vi "TDC_getCoincCounters.vi"(8 "Error In":errorcluster) -> (0 "Error Out":errorcluster, 1 "Update Count":i32, 2 "Penta Coincidences":i32, 3 "Quad Coincidences":i32[](array[numeric]), 5 "Triple Coincidences":i32[](array[numeric]), 7 "Pair Coincidences":i32[](array[numeric]), 11 "Single Counts":i32[](array[numeric]))   [LabVIEW 2011]
uses:
  tdcbase.dll
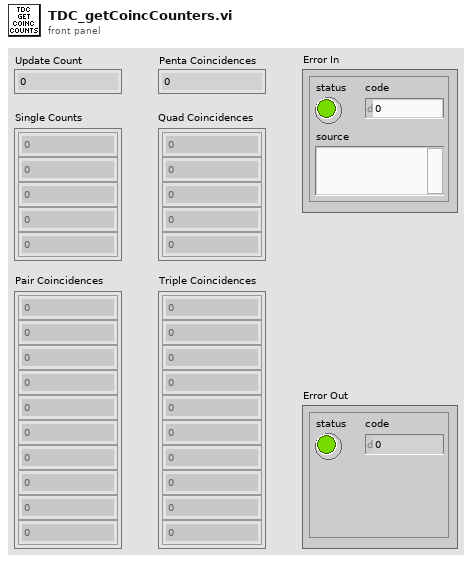
[diagram p1: front panel]
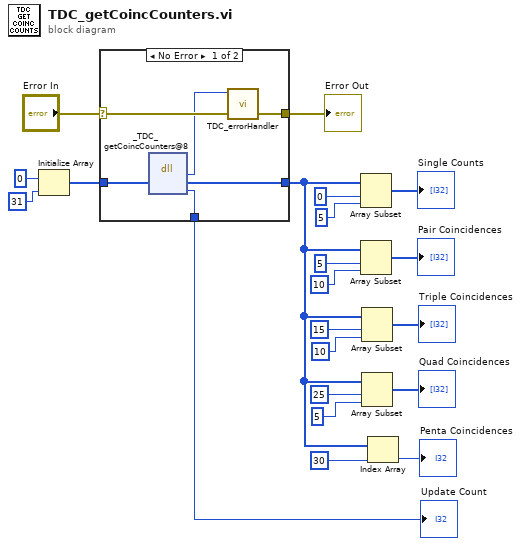
[diagram p0: block diagram]
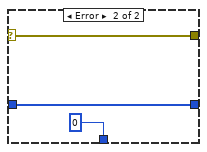
[diagram p2: hidden frame]
diagram:
  n1 = Initialize Array(0, 31) -> (w1:i32[])
  n2 = case shown="No Error" "Error In" {
    selector: "Error In" -> [w26 w30]
    tunnel: [w25 w30] -> w20
    tunnel: [w27 w28] -> w6
    tunnel: [w23 0] -> w4
    tunnel: w1 -> [w22 w28]
    frame No Error {
      n3 = dll-call lib="X:/tdcbase.dll" fn="_TDC_getCoincCounters@8"("data"=w22) -> ("return type"=w24:i32, "data"=w27:i32[], "updates"=w23:i32)  [unwired: 4 in, 2 out]
      n4 = call "TDC_errorHandler.vi"("Error In"=w26, "TDC Return Code"=w24) -> ("Error Out"=w25:errorcluster)  [unwired: 9 in]
    }
    frame Error {
    }
  }
  "Error Out" <- w20
  "Update Count" <- w4
  n5 = Array Subset(array=w6, index=0, length=5) -> (→"Single Counts":i32[])
  n6 = Array Subset(array=w6, index=5, length=10) -> (→"Pair Coincidences":i32[])
  n7 = Array Subset(array=w6, index=15, length=10) -> (→"Triple Coincidences":i32[])
  n8 = Array Subset(array=w6, index=25, length=5) -> (→"Quad Coincidences":i32[])
  n9 = Index Array(array=w6, index=30) -> (element=→"Penta Coincidences":i32)
